vi "flow-icc.vi"(11 "Mode":T1=enum."Off") -> (3 "ICC Flow Templates":T2[](array[typedef]))   [LabVIEW 2024]
uses:
  controls/UiStepBuilder.ctl
  controls/type.step-builder.ctl
  controls/device-mode.ctl
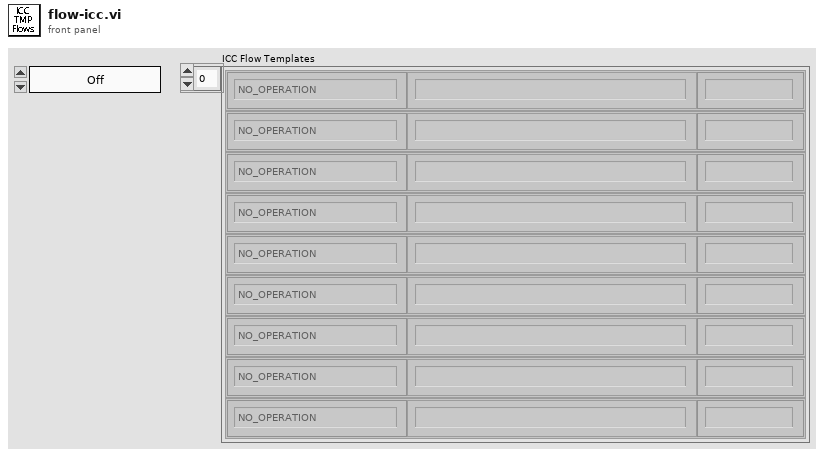
[diagram p1: front panel]
types:
  T1 = typedef "device-mode.ctl" = enum16{"On", "Off", "Sense", "Sched", "Sched AND Sense", "Sched OR Sense"}
  T2 = typedef "UiStepBuilder.ctl" = cluster{"Step Function":T3, "ParamString":string, "Step Label":string}
  T3 = typedef "type.step-builder.ctl" = enum16{"NO_OPERATION", "DELAY-JUMP", "DELAY", "JUMP", "COMPLETE", "SCHEDULER", "IRR-CHECK", "UNIT-CHECK", "UNIT-SAMPLE", "UNIT-DOSE", "LOG-REPORT", "LOG-MESSAGE", "IO-READ", "IO-READ-MANY", "IO-WRITE", "IO-COMPARE-OUT", "IO-COMPARE-IN", "PROC-START", "PROC-STOP", "PROC-LOAD", "PROC-IS-COMPLETED", "RECORD-MOVE", "GET-RH", "GET-UV", "GET-WD", "GET-WS", "OCS-CHECK", "OCS-RECORD"}
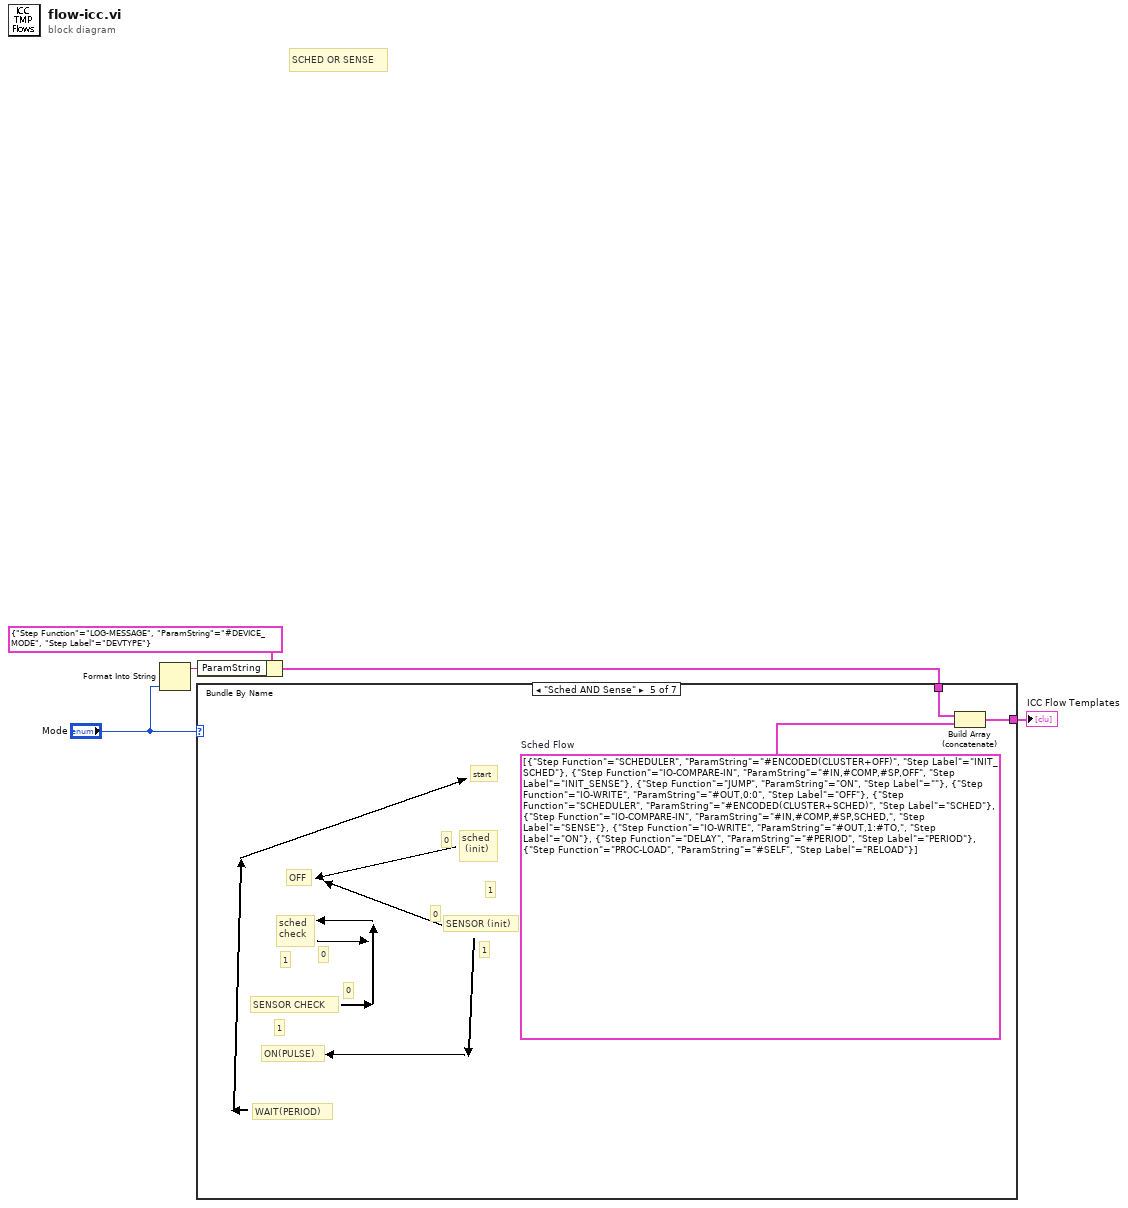
[diagram p0: block diagram]
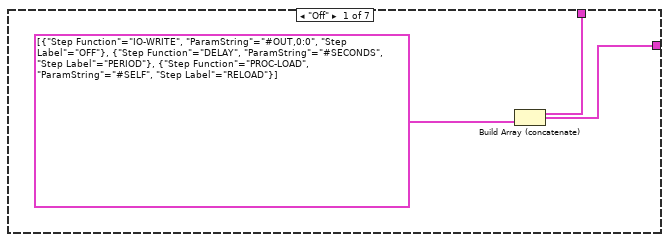
[diagram p2: hidden frame]
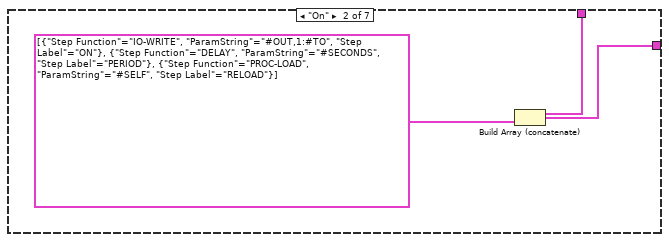
[diagram p3: hidden frame]
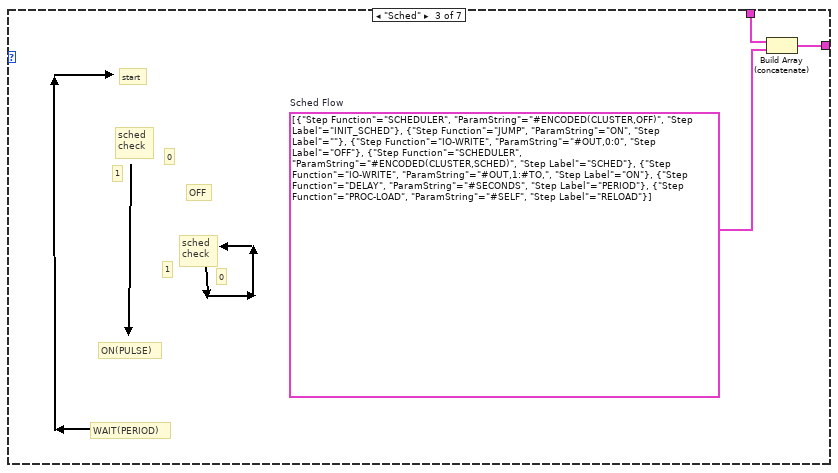
[diagram p4: hidden frame]
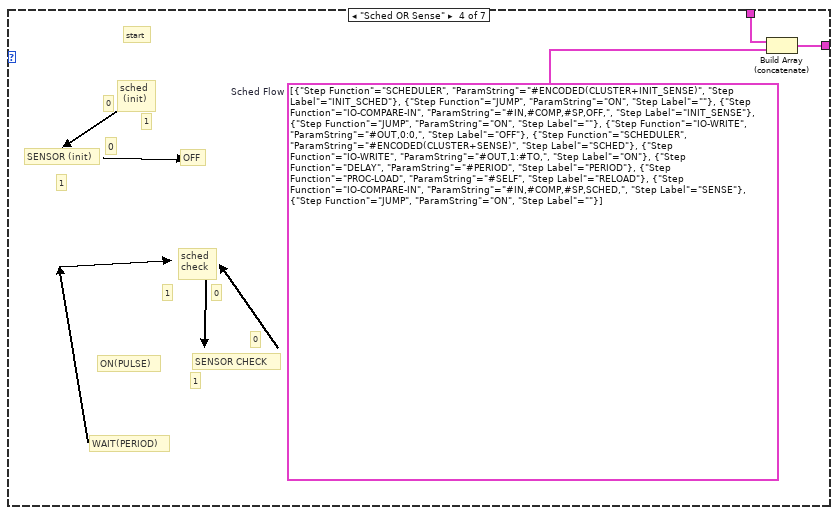
[diagram p5: hidden frame]
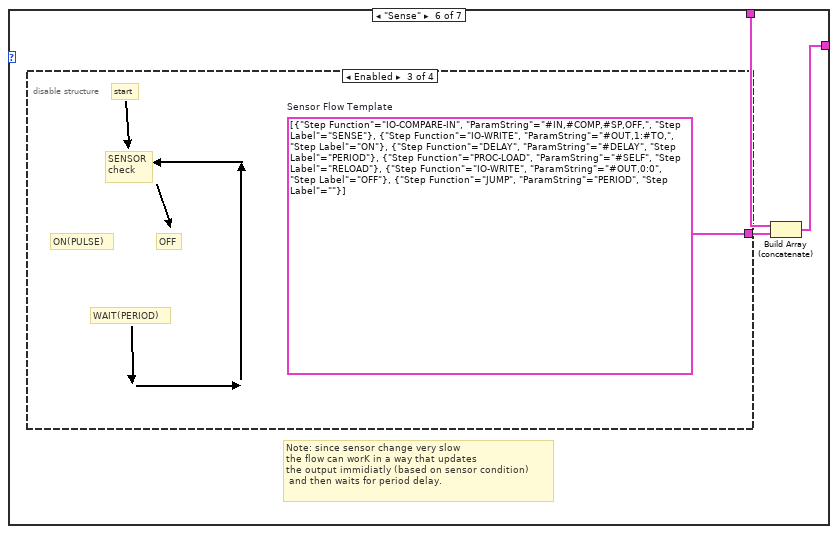
[diagram p6: hidden frame]
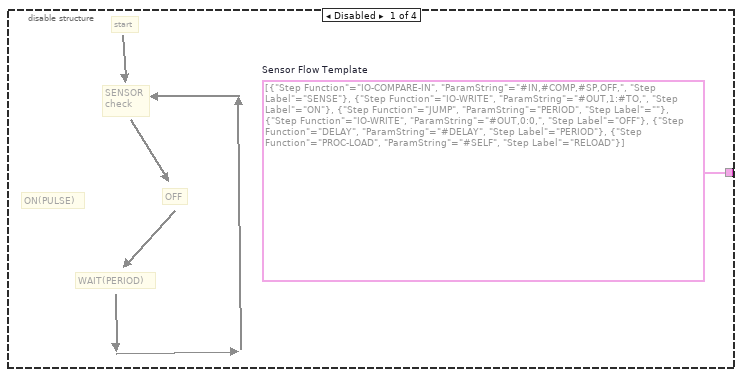
[diagram p7: hidden frame]
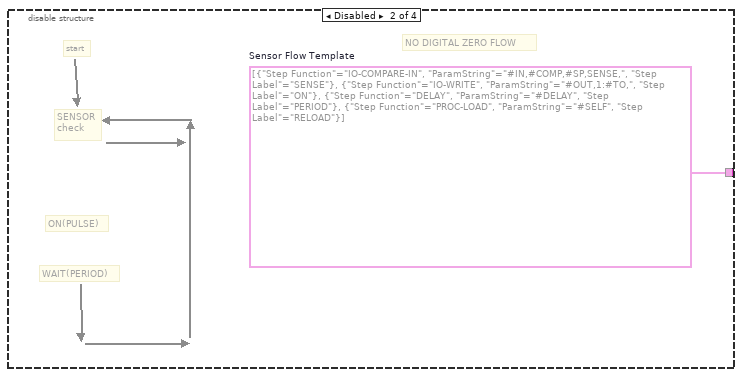
[diagram p8: hidden frame]
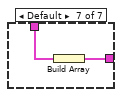
[diagram p10: hidden frame]
diagram:
  # "SCHED OR SENSE"
  n1 = Format Into String("Mode") -> (resulting string=w4:string)  [unwired: 3 in, 1 out]
  n2 = Bundle By Name(cluster=T2 {"Step Function"=enum."LOG-MESSAGE", "ParamString"="#DEVICE_MODE", "Step Label"="DEVTYPE"} ("UiBuilderStep"), "ParamString"=w4) -> (w2:T2)
  n3 = case shown="\"Sched AND Sense\"" "Mode" {
    tunnel: [w6 w9 w13 w16 w19 w22 w27] -> w5
    tunnel: w2 -> [w7 w10 w12 w15 w18 w21 w28]
    frame "Off" {
      n4 = Build Array (concatenate)(w7, T2[] [{"Step Function"=enum."IO-WRITE", "ParamString"="#OUT,0:0", "Step Label"="OFF"}, {"Step Function"=enum."DELAY", "ParamString"="#SECONDS", "Step Label"="PERIOD"}, {"Step Function"=enum."PROC-LOAD", "ParamString"="#SELF", "Step Label"="RELOAD"}] ("UiBuildSteps")) -> (w6:T2[])
    }
    frame "On" {
      n5 = Build Array (concatenate)(w10, T2[] [{"Step Function"=enum."IO-WRITE", "ParamString"="#OUT,1:#TO", "Step Label"="ON"}, {"Step Function"=enum."DELAY", "ParamString"="#SECONDS", "Step Label"="PERIOD"}, {"Step Function"=enum."PROC-LOAD", "ParamString"="#SELF", "Step Label"="RELOAD"}] ("UiBuildSteps")) -> (w9:T2[])
    }
    frame "Sched" {
      w14 = T2[] [{"Step Function"=enum."SCHEDULER", "ParamString"="#ENCODED(CLUSTER,OFF)", "Step Label"="INIT_SCHED"}, {"Step Function"=enum."JUMP", "ParamString"="ON", "Step Label"=""}, {"Step Function"=enum."IO-WRITE", "ParamString"="#OUT,0:0", "Step Label"="OFF"}, {"Step Function"=enum."SCHEDULER", "ParamString"="#ENCODED(CLUSTER,SCHED)", "Step Label"="SCHED"}, {"Step Function"=enum."IO-WRITE", "ParamString"="#OUT,1:#TO,", "Step Label"="ON"}, {"Step Function"=enum."DELAY", "ParamString"="#SECONDS", "Step Label"="PERIOD"}, {"Step Function"=enum."PROC-LOAD", "ParamString"="#SELF", "Step Label"="RELOAD"}]  # Sched Flow
      # "1"
      # "0"
      # "1"
      # "0"
      # "OFF"
      # "sched\ncheck"
      # "start"
      # "WAIT(PERIOD)"
      # "ON(PULSE)"
      # "sched\ncheck"
      n6 = Build Array (concatenate)(w12, w14) -> (w13:T2[])
    }
    frame "Sched OR Sense" {
      w17 = T2[] [{"Step Function"=enum."SCHEDULER", "ParamString"="#ENCODED(CLUSTER+INIT_SENSE)", "Step Label"="INIT_SCHED"}, {"Step Function"=enum."JUMP", "ParamString"="ON", "Step Label"=""}, {"Step Function"=enum."IO-COMPARE-IN", "ParamString"="#IN,#COMP,#SP,OFF,", "Step Label"="INIT_SENSE"}, {"Step Function"=enum."JUMP", "ParamString"="ON", "Step Label"=""}, {"Step Function"=enum."IO-WRITE", "ParamString"="#OUT,0:0,", "Step Label"="OFF"}, {"Step Function"=enum."SCHEDULER", "ParamString"="#ENCODED(CLUSTER+SENSE)", "Step Label"="SCHED"}, {"Step Function"=enum."IO-WRITE", "ParamString"="#OUT,1:#TO,", "Step Label"="ON"}, {"Step Function"=enum."DELAY", "ParamString"="#PERIOD", "Step Label"="PERIOD"}, {"Step Function"=enum."PROC-LOAD", "ParamString"="#SELF", "Step Label"="RELOAD"}, {"Step Function"=enum."IO-COMPARE-IN", "ParamString"="#IN,#COMP,#SP,SCHED,", "Step Label"="SENSE"}, {"Step Function"=enum."JUMP", "ParamString"="ON", "Step Label"=""}]  # Sched Flow
      # "OFF"
      # "1"
      # "0"
      # "1"
      # "0"
      # "SENSOR (init)"
      # "sched \n (init)"
      # "0"
      # "1"
      # "1"
      # "0"
      # "SENSOR CHECK"
      # "start"
      # "WAIT(PERIOD)"
      # "ON(PULSE)"
      # "sched\ncheck"
      n7 = Build Array (concatenate)(w15, w17) -> (w16:T2[])
    }
    frame "Sched AND Sense" {
      w20 = T2[] [{"Step Function"=enum."SCHEDULER", "ParamString"="#ENCODED(CLUSTER+OFF)", "Step Label"="INIT_SCHED"}, {"Step Function"=enum."IO-COMPARE-IN", "ParamString"="#IN,#COMP,#SP,OFF", "Step Label"="INIT_SENSE"}, {"Step Function"=enum."JUMP", "ParamString"="ON", "Step Label"=""}, {"Step Function"=enum."IO-WRITE", "ParamString"="#OUT,0:0", "Step Label"="OFF"}, {"Step Function"=enum."SCHEDULER", "ParamString"="#ENCODED(CLUSTER+SCHED)", "Step Label"="SCHED"}, {"Step Function"=enum."IO-COMPARE-IN", "ParamString"="#IN,#COMP,#SP,SCHED,", "Step Label"="SENSE"}, {"Step Function"=enum."IO-WRITE", "ParamString"="#OUT,1:#TO,", "Step Label"="ON"}, {"Step Function"=enum."DELAY", "ParamString"="#PERIOD", "Step Label"="PERIOD"}, {"Step Function"=enum."PROC-LOAD", "ParamString"="#SELF", "Step Label"="RELOAD"}]  # Sched Flow
      # "1"
      # "1"
      # "OFF"
      # "0"
      # "0"
      # "SENSOR (init)"
      # "sched \n (init)"
      # "1"
      # "0"
      # "1"
      # "0"
      # "SENSOR CHECK"
      # "start"
      # "WAIT(PERIOD)"
      # "ON(PULSE)"
      # "sched\ncheck"
      n8 = Build Array (concatenate)(w18, w20) -> (w19:T2[])
    }
    frame "Sense" {
      # "Note: since sensor change very slow\nthe flow can worK in a way that updates \nthe output immidiatly (based on sensor condition)\n and then waits for period delay."
      n9 = disable-structure shown="Enabled" {
        disable-tunnel: [w24 w25 w26 _] -> w23
        frame Disabled {
          w24 = T2[] [{"Step Function"=enum."IO-COMPARE-IN", "ParamString"="#IN,#COMP,#SP,OFF,", "Step Label"="SENSE"}, {"Step Function"=enum."IO-WRITE", "ParamString"="#OUT,1:#TO,", "Step Label"="ON"}, {"Step Function"=enum."JUMP", "ParamString"="PERIOD", "Step Label"=""}, {"Step Function"=enum."IO-WRITE", "ParamString"="#OUT,0:0,", "Step Label"="OFF"}, {"Step Function"=enum."DELAY", "ParamString"="#DELAY", "Step Label"="PERIOD"}, {"Step Function"=enum."PROC-LOAD", "ParamString"="#SELF", "Step Label"="RELOAD"}]  # Sensor Flow Template
          # "start"
          # "WAIT(PERIOD)"
          # "OFF"
          # "ON(PULSE)"
          # "SENSOR\ncheck"
        }
        frame Disabled {
          w25 = T2[] [{"Step Function"=enum."IO-COMPARE-IN", "ParamString"="#IN,#COMP,#SP,SENSE,", "Step Label"="SENSE"}, {"Step Function"=enum."IO-WRITE", "ParamString"="#OUT,1:#TO,", "Step Label"="ON"}, {"Step Function"=enum."DELAY", "ParamString"="#DELAY", "Step Label"="PERIOD"}, {"Step Function"=enum."PROC-LOAD", "ParamString"="#SELF", "Step Label"="RELOAD"}]  # Sensor Flow Template
          # "start"
          # "WAIT(PERIOD)"
          # "ON(PULSE)"
          # "SENSOR\ncheck"
          # "NO DIGITAL ZERO FLOW"
        }
        frame Enabled {
          w26 = T2[] [{"Step Function"=enum."IO-COMPARE-IN", "ParamString"="#IN,#COMP,#SP,OFF,", "Step Label"="SENSE"}, {"Step Function"=enum."IO-WRITE", "ParamString"="#OUT,1:#TO,", "Step Label"="ON"}, {"Step Function"=enum."DELAY", "ParamString"="#DELAY", "Step Label"="PERIOD"}, {"Step Function"=enum."PROC-LOAD", "ParamString"="#SELF", "Step Label"="RELOAD"}, {"Step Function"=enum."IO-WRITE", "ParamString"="#OUT,0:0", "Step Label"="OFF"}, {"Step Function"=enum."JUMP", "ParamString"="PERIOD", "Step Label"=""}]  # Sensor Flow Template
          # "start"
          # "OFF"
          # "WAIT(PERIOD)"
          # "ON(PULSE)"
          # "SENSOR\ncheck"
        }
        frame Disabled {
        }
      }
      n10 = Build Array (concatenate)(w21, w23) -> (w22:T2[])
    }
    frame Default {
      n11 = Build Array(w28) -> (w27:T2[])
    }
  }
  "ICC Flow Templates" <- w5
